vi "Apply UI State.vi"(5 "Ctls Refs (All Ctls)":refnum<vi>[](array[refnum]), 6 "Traverse Clusters (F)":bool, 7 "VI Ref (Calling VI)":refnum<vi>, 8 "Error In":errorcluster, 10 "State Name":string, 11 "UIM In":refnum<data-value>) -> (0 "Error Out":errorcluster, 3 "UIM Out":refnum<data-value>)   [LabVIEW 2020, in "UIM.lvlib" / "UIM.lvclass"]
doc: "Apply the previously saved UI state to controls and indicators of the calling VI. \n\n<b>VI Ref (Calling VI) -</b> Allows you to point to the VI you want to work with. If the VI Ref is left unwired the calling VI reference will be used. \n\n<b>Ctls Refs (All Ctls) -</b> If the Ctls Refs are unwired, all control references and their properties, handled by UIPs in the UIM, will be captured to the state definition. By wiring this input you can optimize the performance of this method, because it will not need to traverse and obtain references to all controls and indicators of a VIs front panel.\n\n<b>Travers Clusters -</b> Defines if the clusters are considered compound controls, disposing their contents, or not. Use this if you want to capture the UIPs on the controls inside of clusters."
uses:
  UIM.lvclass
  UIM.lvclass/UIM.ctl
  UIP Interface/UIP Interface.lvclass
  <vilib>/Utility/LVClass/Get LV Class Name.vi
  <vilib>/Utility/error.llb/Error Cluster From Error Code.vi
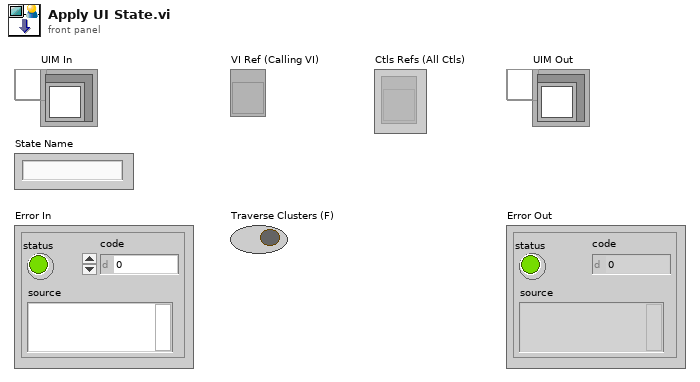
[diagram p1: front panel]
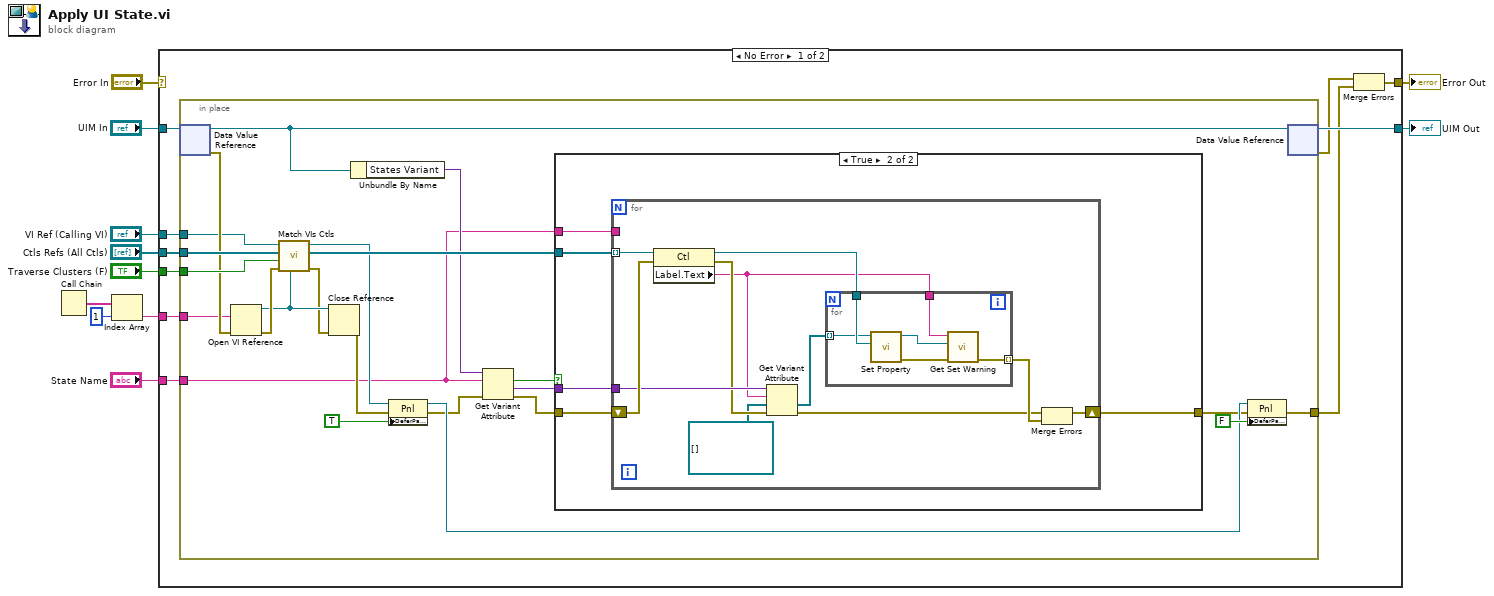
[diagram p0: block diagram]
diagram:
  n1 = Call Chain() -> (call chain=w3:string[])
  n2 = Index Array(array=w3, index=1) -> (element=w2:string)
  n3 = case shown="No Error" "Error In" {
    selector: "Error In" -> [_ w69]
    tunnel: "UIM In" -> [w21 w68]
    tunnel: [w20 w68] -> w10
    tunnel: "State Name" -> [w19 _]
    tunnel: "Ctls Refs (All Ctls)" -> [w18 _]
    tunnel: "VI Ref (Calling VI)" -> [w17 _]
    tunnel: "Traverse Clusters (F)" -> [w16 _]
    tunnel: [w15 w69] -> w5
    tunnel: w2 -> [w12 _]
    frame No Error {
      n4 = in-place {
        in-place-border: [w33] -> w14
        in-place-border: w19 -> [w29]
        in-place-border: w18 -> [w42]
        in-place-border: w17 -> [w24]
        in-place-border: w16 -> [w32]
        in-place-border: w12 -> [w23]
        n5 = in-place-dvr #1(w21) -> (w44:refnum<class "UIM.lvclass">, w31:errorcluster)
        n6 = Open VI Reference(vi path=w23, error in (no error)=w31) -> (vi reference=w39:refnum<vi>, error out=w43:errorcluster)  [unwired: 4 out]
        n7 = call "Match VIs Ctls.vi"("Calling VI Ref"=w39, "Error In"=w43, "Traverse Clusters (F)"=w32, "Ctls Refs (All Ctls)"=w42, "VI Ref"=w24) -> ("Error Out"=w38:errorcluster, "Matching Ctls Out"=w41:refnum<vi>[], "Used Panel"=w40:refnum<vi>)  [unwired: 4 in]
        n8 = Close Reference(reference=w39, error in (no error)=w38) -> (error out=w37:errorcluster)
        n9 = Unbundle By Name(w44) -> ("States Variant"=w30:variant)
        n10 = property class="Pnl"(reference=w40, error in=w37, "DeferPanUpdts"=TRUE ("Defer Panel Updates")) -> (reference out=w34:refnum<vi>, error out=w28:errorcluster)
        n11 = Get Variant Attribute(Variant=w30, name=w29, error in=w28) -> (found=w27:bool, value=w26:variant, error out=w25:errorcluster)  [unwired: 1 in, 1 out]
        n12 = case shown="True" w27 {
          tunnel: w25 -> [w45 w47]
          tunnel: w41 -> [_ w50]
          tunnel: w29 -> [_ w49]
          tunnel: w26 -> [_ w48]
          tunnel: [w45 w46] -> w22
          frame False {
          }
          frame True {
            n13 = for {
              tunnel: w50 -> [w61] mode=indexing
              tunnel: w48 -> [w57]
              shift-right: [w52] -> w46
              shift-left: w47 -> [w60]
              tunnel: w49 -> [_]
              n14 = property class="Ctl"(reference=w61, error in=w60) -> (reference out=w59:refnum<vi>, error out=w56:errorcluster, "Label.Text"=w51:string)
              n15 = Get Variant Attribute(Variant=w57, name=w51, default value (empty Variant)=refnum<class "UIP Interface.lvclass">[] [] ("UIP Defs"), error in=w56) -> (value=w54:refnum<class "UIP Interface.lvclass">[], error out=w53:errorcluster)  [unwired: 2 out]
              n16 = for {
                tunnel: w54 -> [w66] mode=indexing
                tunnel: w59 -> [w67]
                tunnel: [w64] -> w58 mode=indexing
                tunnel: w51 -> [w63]
                n17 = call-dynamic "Set Property.vi"("Ctl Ref"=w67, "UIP In"=w66) -> ("Error Out"=w62:errorcluster, "UIP Out"=w65:refnum<class "UIP Interface.lvclass">)  [unwired: 8 in]
                n18 = call "Get Set Warning.vi"("Error In"=w62, "UIP"=w65, "Label.Text"=w63) -> ("Error Out"=w64:errorcluster)  [unwired: 8 in]
              }
              n19 = Merge Errors(w53, w58) -> (w52:errorcluster)
            }
          }
        }
        n20 = property class="Pnl"(reference=w34, error in=w22, "DeferPanUpdts"=FALSE ("Defer Panel Updates")) -> (error out=w33:errorcluster)  [unwired: 1 out]
        n21 = in-place-dvr #1(w44) -> (w20:refnum<data-value>, w13:errorcluster)
      }
      n22 = Merge Errors(w13, w14) -> (w15:errorcluster)
    }
    frame Error {
    }
  }
  "UIM Out" <- w10
  "Error Out" <- w5
